vi "VI Tree - string__ogtk.vi"   [LabVIEW 2018]
uses:
  <userlib>/_OpenG.lib/string/string.llb/Trim Whitespace (String)__ogtk.vi
  <userlib>/_OpenG.lib/string/string.llb/Convert EOLs (String)__ogtk.vi
  <userlib>/_OpenG.lib/string/string.llb/To Proper Case (String)__ogtk.vi
  <userlib>/_OpenG.lib/string/string.llb/To Camel Case (String)__ogtk.vi
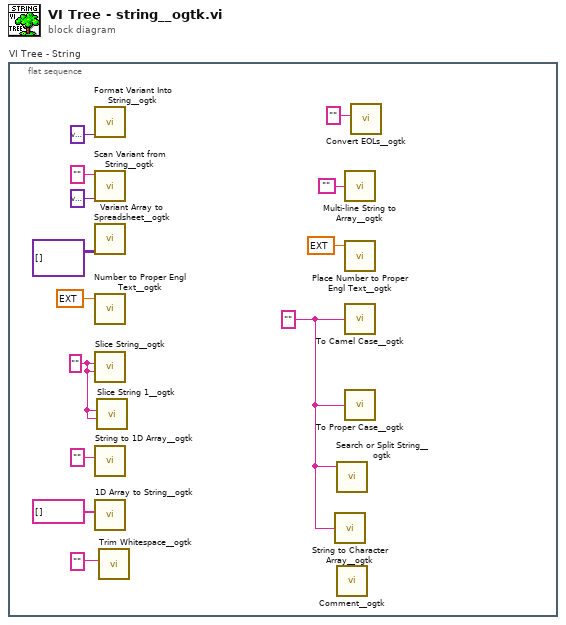
[diagram p0: block diagram]
diagram:
  n1 = flat-sequence "VI Tree - String" {
    frame #0 {
      w1 = "" ("string")
      w2 = "" ("string")
      n2 = call <userlib>:"Format Variant Into String__ogtk.vi"("Variant"=variant) -> ()  [unwired: 13 in, 2 out]
      n3 = call <userlib>:"Scan Variant from String__ogtk.vi"("Default Value"=variant, "Input String"="") -> ()  [unwired: 6 in, 4 out]
      n4 = call <userlib>:"Variant Array to Spreadsheet__ogtk.vi"("2D Variant Array"=variant[][] []) -> ()  [unwired: 9 in, 2 out]
      n5 = call <userlib>:"Number to Proper Engl Text__ogtk.vi"("Numeric"=ext 0.0) -> ()  [unwired: 4 in, 1 out]
      n6 = call <userlib>:"Slice String__ogtk.vi"("slice"=w2, "string"=w2) -> ()  [unwired: 5 in, 1 out]
      n7 = call <userlib>:"String to 1D Array__ogtk.vi"("string"="") -> ()  [unwired: 10 in, 1 out]
      n8 = call <userlib>:"1D Array to String__ogtk.vi"("Array of Strings"=string[] []) -> ()  [unwired: 10 in, 1 out]
      n9 = call <userlib>:"Slice String 1__ogtk.vi"("Subset (i:j)"=w2, "String"=w2) -> ()  [unwired: 7 in, 1 out]
      n10 = call-poly <userlib>:"Trim Whitespace__ogtk.vi"("String in"="") -> ()  [unwired: 6 in, 1 out]
      n11 = call <userlib>:"String to Character Array__ogtk.vi"("Input String"=w1) -> ()  [unwired: 1 out]
      n12 = call <userlib>:"Search or Split String__ogtk.vi"("string"=w1) -> ()  [unwired: 2 in, 3 out]
      n13 = call <userlib>:"Comment__ogtk.vi"() -> ()  [unwired: 1 in]
      n14 = call <userlib>:"Multi-line String to Array__ogtk.vi"("string"="") -> ()  [unwired: 1 out]
      n15 = call <userlib>:"Place Number to Proper Engl Text__ogtk.vi"("Numeric"=ext 0.0) -> ()  [unwired: 4 in, 1 out]
      n16 = call-poly <userlib>:"To Camel Case__ogtk.vi"("string"=w1) -> ()  [unwired: 1 in, 1 out]
      n17 = call-poly <userlib>:"To Proper Case__ogtk.vi"("string"=w1) -> ()  [unwired: 4 in, 1 out]
      n18 = call-poly <userlib>:"Convert EOLs__ogtk.vi"("String in"="") -> ()  [unwired: 10 in, 1 out]
    }
  }
